vi "Get LTS Max Stage Acceleration.vi"(8 "error in (no error)":errorcluster, 10 "Cluster in":T1, 11 "LTS Reference In":refnum<k24>) -> (0 "error out":errorcluster, 1 "AccelerationMaximum":dbl, 2 "Cluster out":T1, 3 "LTS Reference Out":refnum<k24>, 4 "VelocityMaximum":dbl)   [LabVIEW 2018]
uses:
  Controls/Translation Stage Cluster.ctl
  General/Controls/Translation Stage Types.ctl
  C:/Project/SerialSectOCT - FFT GPU/SerialSectOCT/Labview Software/Thorlabs.MotionControl.Controls.dll
  Thorlabs.MotionControl.Controls.dll
  C:/Project/SerialSectOCT - FFT GPU/SerialSectOCT/Labview Software/Thorlabs.MotionControl.IntegratedStepperMotorsCLI.dll
  Thorlabs.MotionControl.IntegratedStepperMotorsCLI.dll
  C:/Project/SerialSectOCT - FFT GPU/SerialSectOCT/Labview Software/Thorlabs.MotionControl.GenericMotorCLI.dll
  Thorlabs.MotionControl.GenericMotorCLI.dll
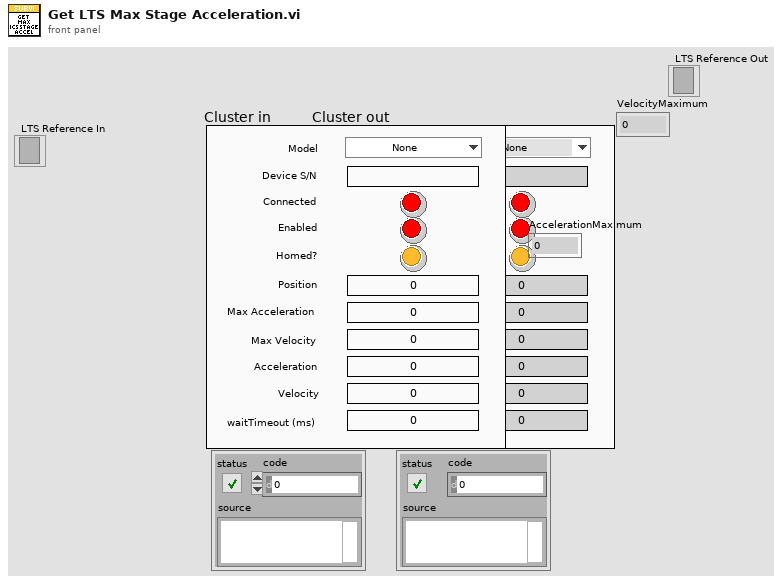
[diagram p1: front panel]
types:
  T1 = typedef "Translation Stage Cluster.ctl" = cluster{"Position":dbl, "Is.Enabled?":bool, "Is.Connected?":bool, "Device SN":string, "AccelerationMaximum":dbl, "VelocityMaximum":dbl, "Acceleration":dbl, "Velocity":dbl, "waitTimeout (ms)":i32, "Model":T2, "Is.Homed?":bool}
  T2 = typedef "Translation Stage Types.ctl" = enum16{"None", "Thorlabs LTS", "Thorlabs MLJ"}
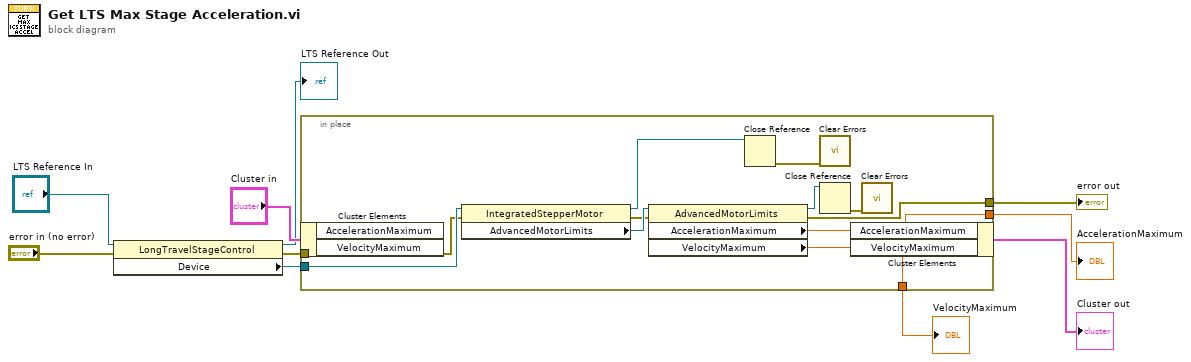
[diagram p0: block diagram]
diagram:
  n1 = property class="LongTravelStageControl"(reference="LTS Reference In", error in="error in (no error)") -> (reference out=→"LTS Reference Out":refnum<k24>, error out=w5:errorcluster, "Device"=w2:refnum<k24>)
  n2 = in-place {
    in-place-border: [w15] -> w8
    in-place-border: w2 -> [w14]
    in-place-border: w5 -> [w13]
    in-place-border: [w12] -> w7
    in-place-border: [w11] -> w1
    n3 = in-place-cluster #1("Cluster in") -> ()  [unwired: 2 out]
    n4 = property class="IntegratedStepperMotor"(reference=w14, error in=w13) -> (reference out=w18:refnum<k24>, error out=w20:errorcluster, "AdvancedMotorLimits"=w21:refnum<k24>)
    n5 = property class="AdvancedMotorLimits"(reference=w21, error in=w20) -> (reference out=w16:refnum<k24>, error out=w15:errorcluster, "AccelerationMaximum"=w12:dbl, "VelocityMaximum"=w11:dbl)
    n6 = Close Reference(reference=w18) -> (error out=w19:errorcluster)  [unwired: 1 in]
    n7 = call <vilib>:"Clear Errors.vi"("error in (no error)"=w19) -> ()  [unwired: 5 in, 2 out]
    n8 = Close Reference(reference=w16) -> (error out=w17:errorcluster)  [unwired: 1 in]
    n9 = in-place-cluster #1("AccelerationMaximum"=w12, "VelocityMaximum"=w11) -> (→"Cluster out":T1)
    n10 = call <vilib>:"Clear Errors.vi"("error in (no error)"=w17) -> ()  [unwired: 5 in, 2 out]
  }
  "error out" <- w8
  "AccelerationMaximum" <- w7
  "VelocityMaximum" <- w1
